vi "heartbeat.vi"(8 "error in (no error)":errorcluster) -> (0 "error out":errorcluster)   [LabVIEW 2014]
uses:
  Controls/Heartbeat Message.ctl
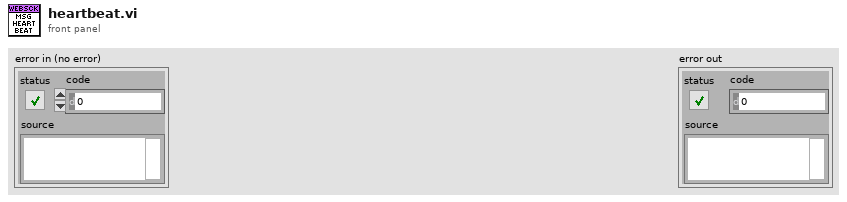
[diagram p1: front panel]
types:
  T1 = typedef "Heartbeat Message.ctl" = cluster{"heartbeat":u8}
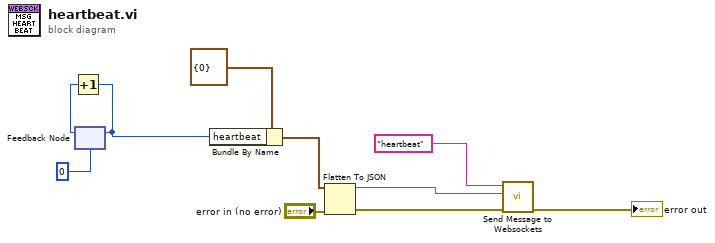
[diagram p0: block diagram]
diagram:
  n1 = feedback #1(u8 0) -> (w9:u8)
  n2 = Increment(x=w9) -> (x+1=w7:u8)
  n3 = feedback-in #1(w7) -> ()
  n4 = Bundle By Name(cluster=T1 {"heartbeat"=0} ("heartbeat"), "heartbeat"=w7) -> (w6:T1)
  n5 = Flatten To JSON(anything=w6, error in (no error)="error in (no error)") -> (JSON string=w3:string, 11:w4:errorcluster)  [unwired: 1 in]
  n6 = call "Send Message to Websockets.vi"("Error In"=w4, "Data"=w3, "Command"="heartbeat") -> ("error out"=→"error out":errorcluster)  [unwired: 8 in]
